vi "Configuration Window.vi"(8 "error in (no error)":errorcluster, 11 "Inst.RP100 in":refnum<class "Inst.RP100.lvclass">) -> (0 "error out":errorcluster, 3 "Inst.RP100 out":refnum<class "Inst.RP100.lvclass">)   [LabVIEW 2019, in "Inst.RP100.lvlib" / "Inst.RP100.lvclass"]
uses:
  Inst.RP100.lvclass
  C:/Program Files (x86)/National Instruments/LabVIEW 2019/user.lib/LevyLab/Instrument Framework/Instrument/Instrument.lvclass
  <userlib>/LevyLab/Instrument Framework/Instrument/Instrument.lvclass/Instrument.ctl
  <userlib>/LevyLab/Instrument Framework/Instrument/Instrument.lvclass
  C:/Program Files (x86)/National Instruments/LabVIEW 2019/user.lib/LevyLab/Instrument Framework/Instrument Types/Strain/Instrument.Strain.lvclass
  C:/Program Files (x86)/National Instruments/LabVIEW 2019/vi.lib/JKI/JKI SMO/SMO/SMO.lvclass
panel:
  in  "Cancel":bool
  in  "RP100 Address":refnum<visa-resource-name>
  in  "OK":bool
  # "Confirm or Make Changes:"
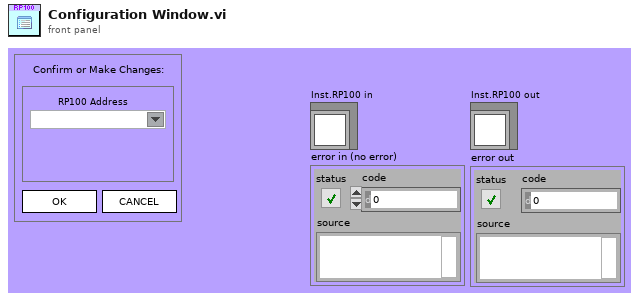
[diagram p1: front panel]
types:
  T1 = enum32{"Invalid", "Standard", "Closed", "Hidden", "Minimized", "Maximized"}
  T2 = enum32{"invalid app kind", "Development System", "Run Time System", "Student Edition", "Embedded LabVIEW", "Evaluation", "Custom"}
  T3 = cluster{"Core":cluster{"Current VI Reference":refnum<vi>, "Close Panel on Exit?":bool}, "Address":string}
  T4 = cluster{"Current VI Reference":refnum<vi>, "Close Panel on Exit?":bool}
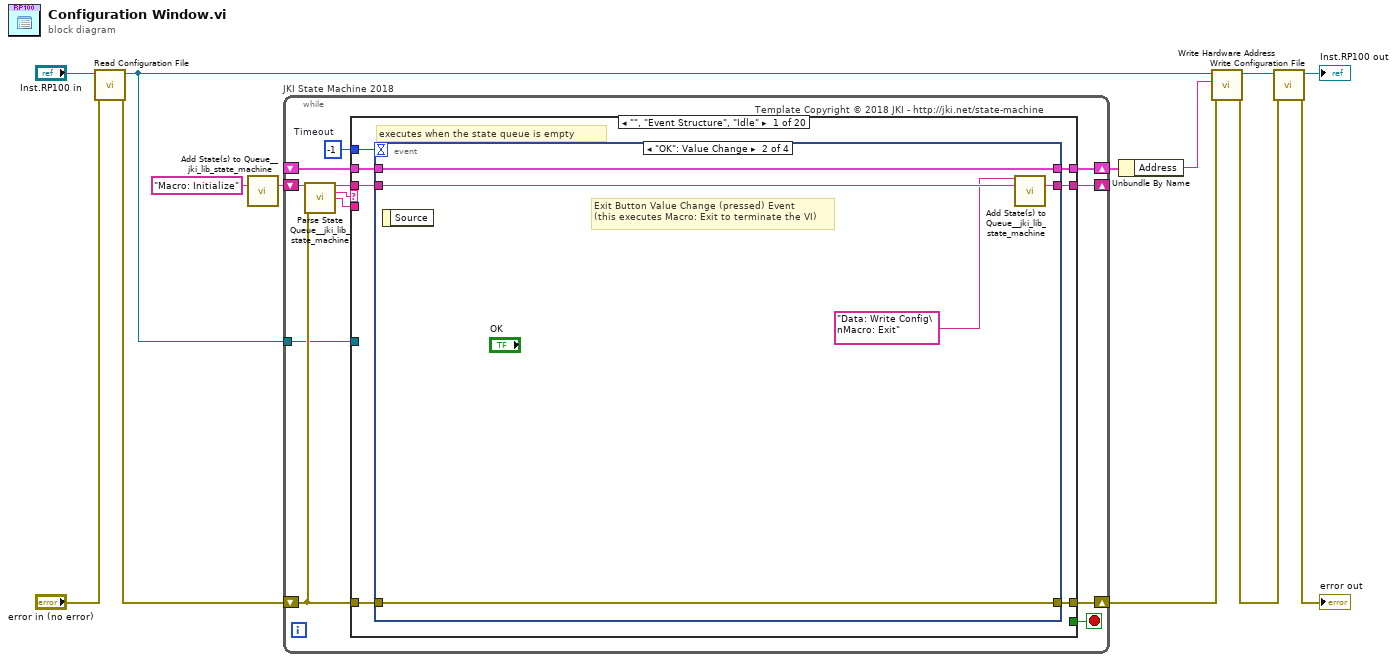
[diagram p0: block diagram]
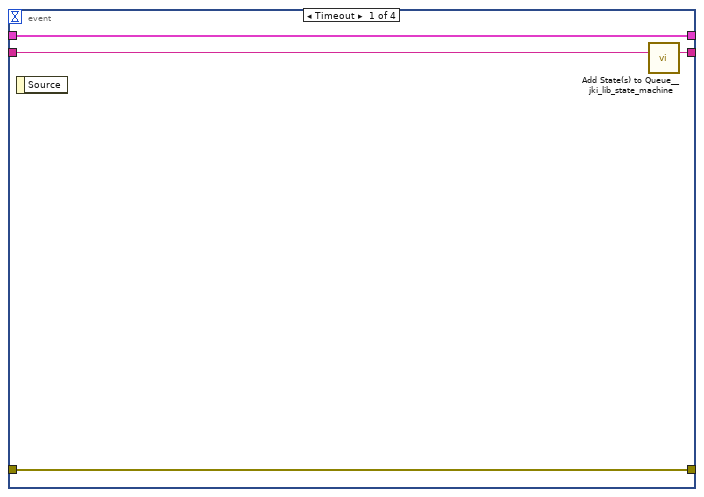
[diagram p2: hidden frame]
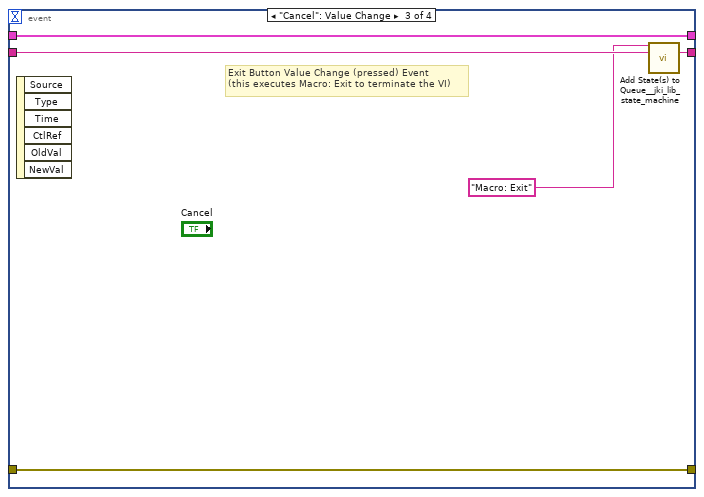
[diagram p3: hidden frame]
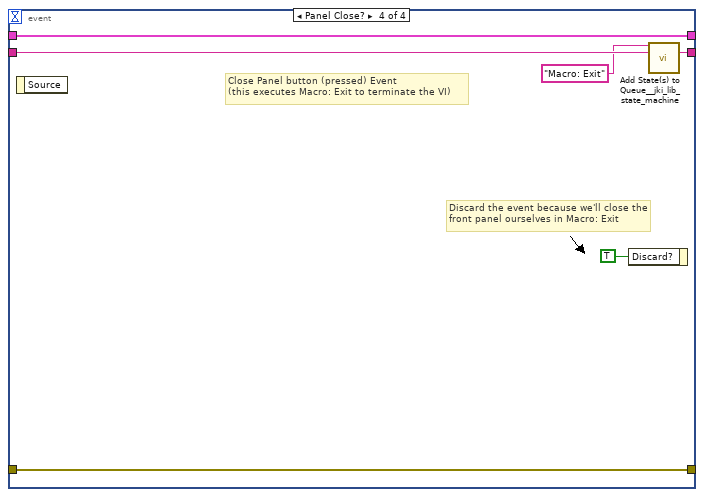
[diagram p4: hidden frame]
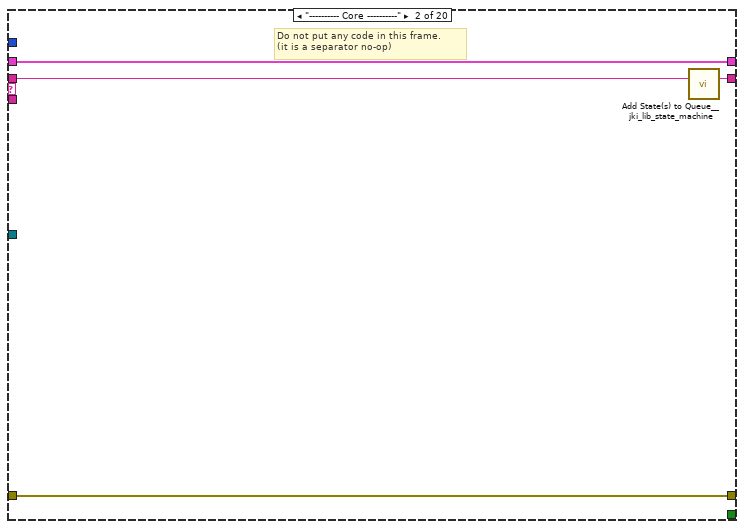
[diagram p5: hidden frame]
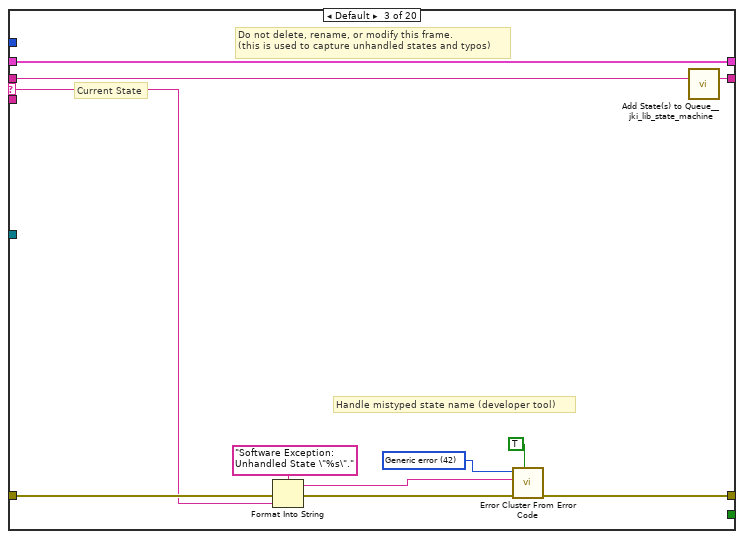
[diagram p6: hidden frame]
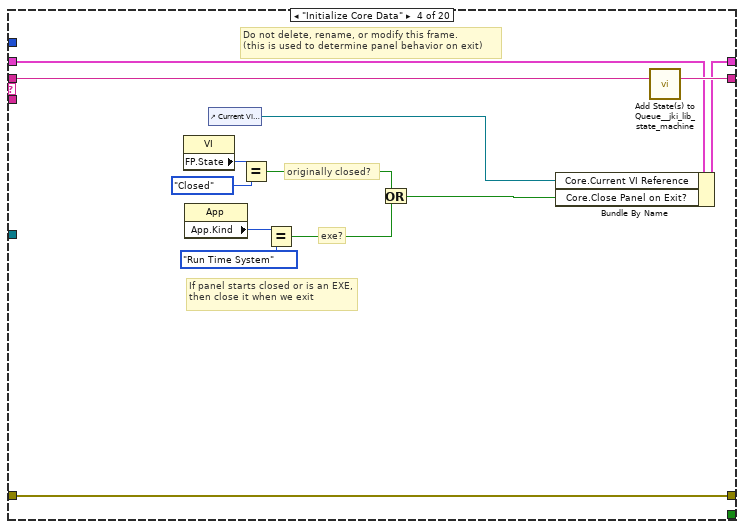
[diagram p7: hidden frame]
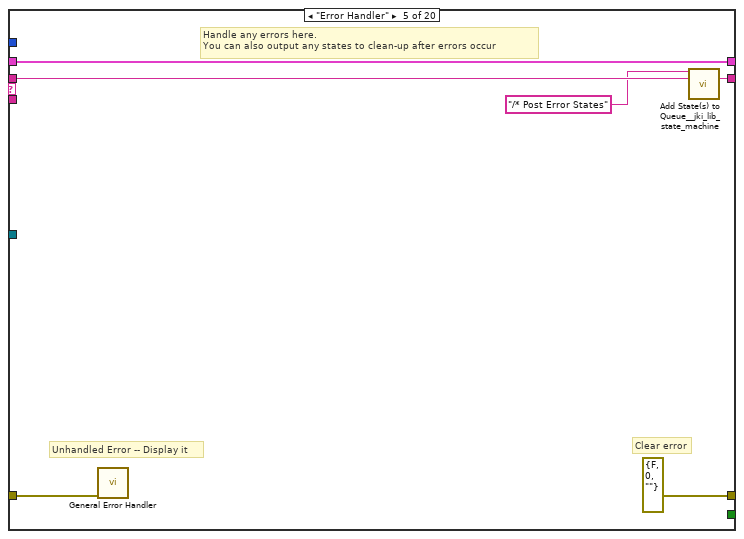
[diagram p8: hidden frame]
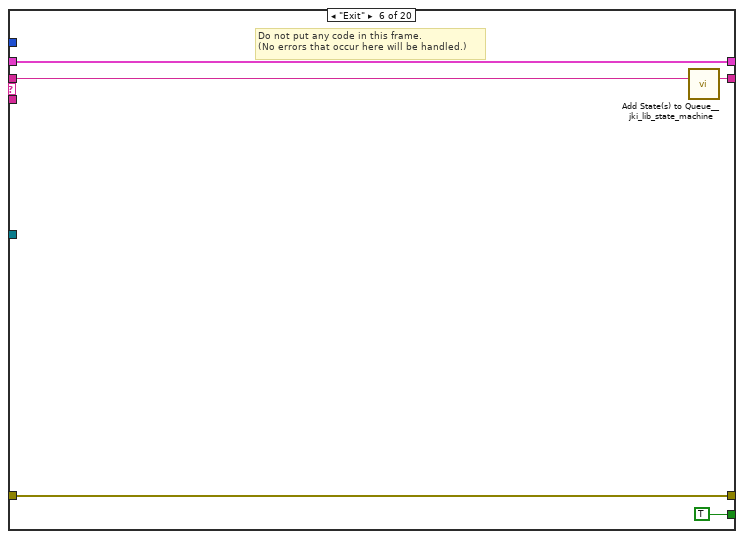
[diagram p9: hidden frame]
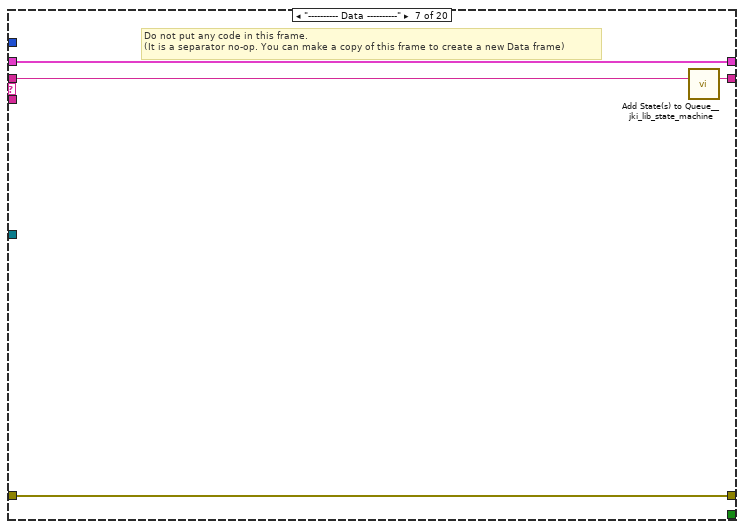
[diagram p10: hidden frame]
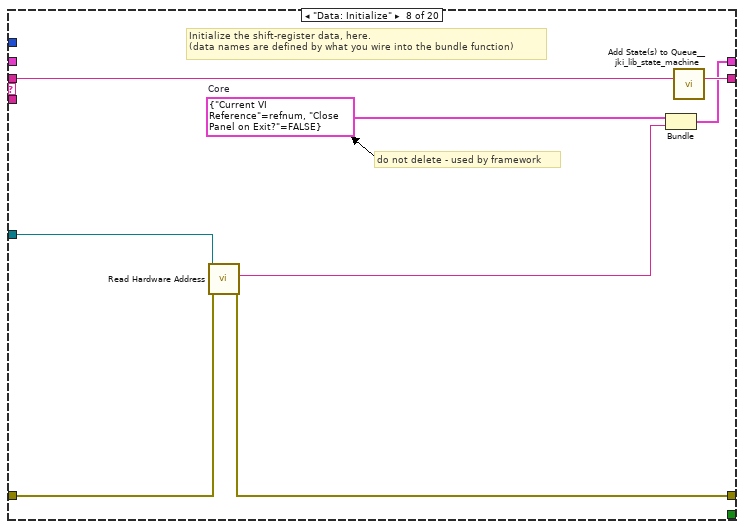
[diagram p11: hidden frame]
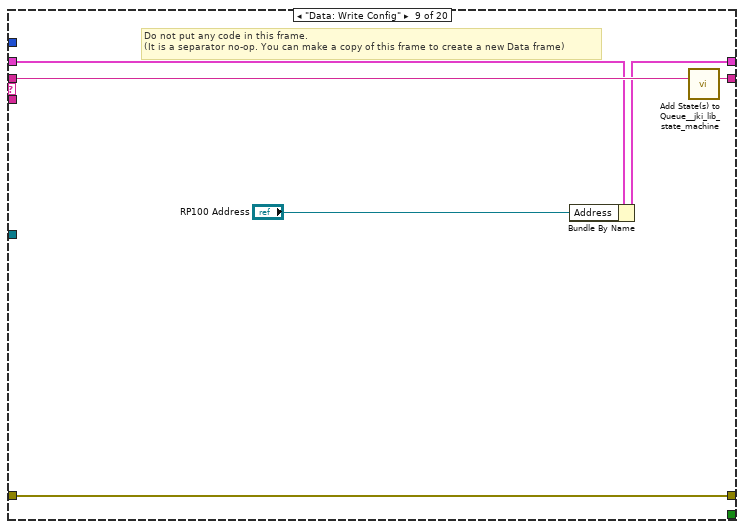
[diagram p12: hidden frame]
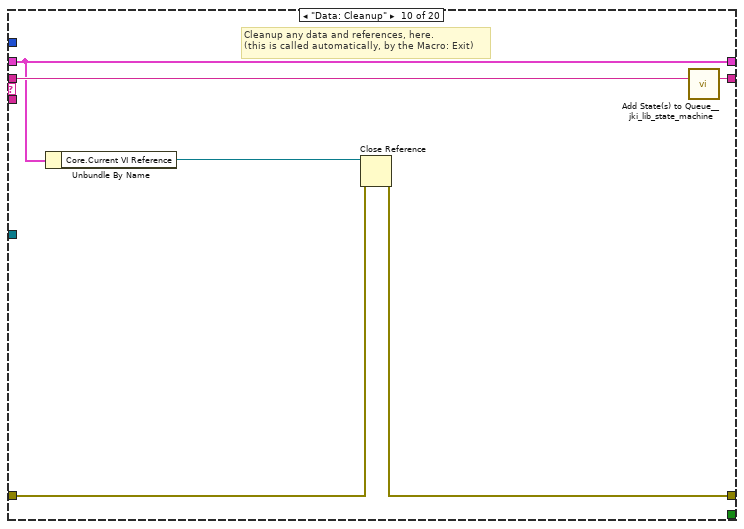
[diagram p13: hidden frame]
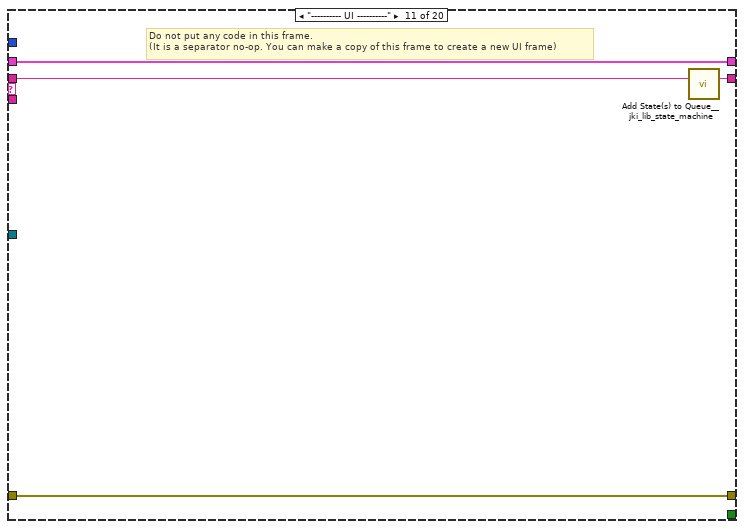
[diagram p14: hidden frame]
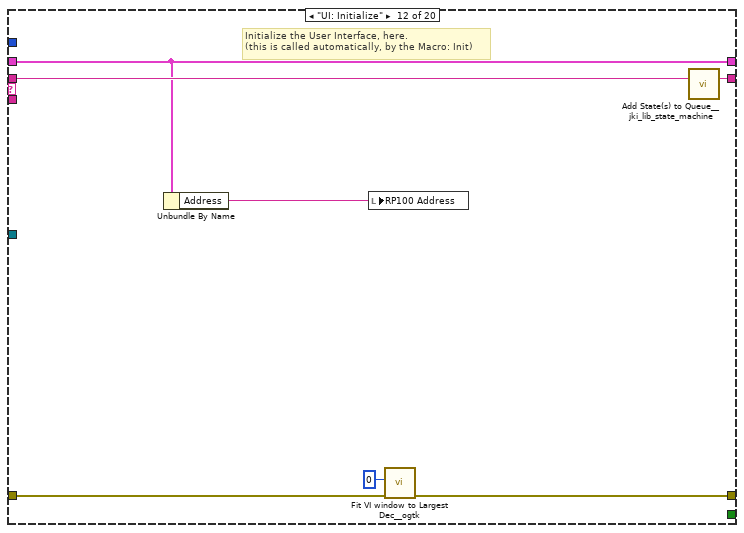
[diagram p15: hidden frame]
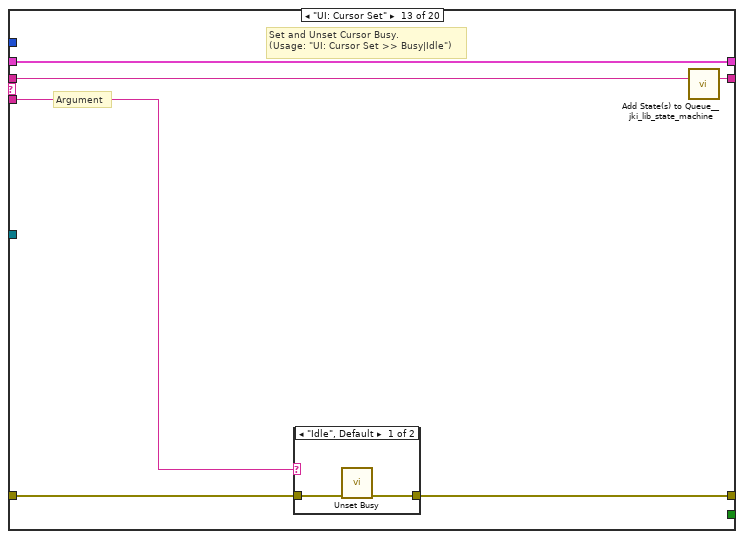
[diagram p16: hidden frame]
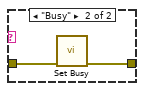
[diagram p17: hidden frame]
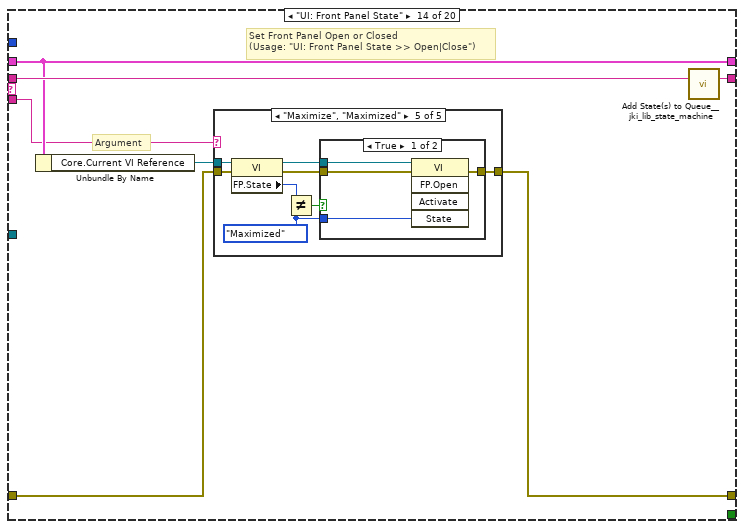
[diagram p18: hidden frame]
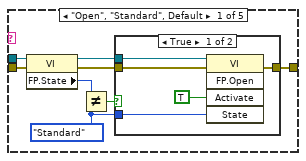
[diagram p19: hidden frame]
diagram:
  n1 = call-dynamic "Read Configuration File.vi"("error in (no error)"="error in (no error)", "Inst.RP100 in"="Inst.RP100 in") -> ("error out"=w8:errorcluster, "Inst.RP100 out"=w6:refnum<class "Inst.RP100.lvclass">)  [unwired: 8 in]
  n2 = call <vilib>:"Add State(s) to Queue__jki_lib_state_machine.vi"("State(s) in (\"\")"="Macro: Initialize") -> ("States Out"=w13:string)  [unwired: 14 in]
  n3 = while "JKI State Machine 2018" {
    shift-right: [w18] -> w2
    shift-left: _ -> [w17]
    shift-right: [w21] -> w4
    shift-left: w8 -> [w15]
    shift-right: [w20] -> _
    shift-left: w13 -> [w22]
    tunnel: w6 -> [w14]
    stop <- w19 stop-if-true
    w16 = -1  # Timeout
    # "Template Copyright © 2018 JKI - http://jki.net/state-machine"
    n4 = call <vilib>:"Parse State Queue__jki_lib_state_machine.vi"("State Queue"=w22, "Error In (no error)"=w15) -> ("Remaining States"=w24:string, "Current State"=w25:string, "Arguments"=w23:string)  [unwired: 11 in]
    n5 = case shown="\"\", \"Event Structure\", \"Idle\"" w25 {
      selector: w25 -> [_ _ w57 _ _ _ _ _ _ _ _ _ _ _ _ _ _ _ _ _]
      tunnel: w24 -> [w32 w56 w61 w80 w86 w91 w95 w103 w109 w115 w119 w126 w132 w143 w212 w217 w227 w231 w235 w239]
      tunnel: w23 -> [_ _ _ _ _ _ _ _ _ _ _ _ w127 w137 _ _ _ _ _ _]
      tunnel: w17 -> [w30 w53 w59 w73 w83 w89 w92 _ w106 w110 w116 w121 w130 w139 w209 w214 w224 w228 w232 w236]
      tunnel: [w29 w54 w63 w77 errorcluster {"status"=FALSE, "code"=0, "source"=""} ("error out") w88 w93 w97 w104 w111 w117 w124 w128 w140 w210 w215 w225 w229 w233 w237] -> w21
      tunnel: w15 -> [w28 w54 w62 w77 w82 w88 w93 w96 w104 w112 w117 w123 w129 w141 w210 w215 w225 w229 w233 w237]
      tunnel: [w31 w55 w60 w79 w85 w90 w94 w102 w108 w114 w118 w125 w131 w142 w211 w216 w226 w230 w234 w238] -> w20
      tunnel: [_ _ _ _ _ TRUE _ _ _ _ _ _ _ _ _ _ _ _ _ _] -> w19
      tunnel: [w27 w53 w59 w78 w83 w89 w92 w101 w107 w110 w116 w121 w130 w139 w209 w214 w224 w228 w232 w236] -> w18
      tunnel: w16 -> [w26 _ _ _ _ _ _ _ _ _ _ _ _ _ _ _ _ _ _ _]
      tunnel: w14 -> [_ _ _ _ _ _ _ w99 _ _ _ _ _ _ _ _ _ _ _ _]
      frame "", "Event Structure", "Idle" {
        # "executes when the state queue is empty"
        n6 = event shown="[1] \"OK\": Value Change" {
          selector: _ -> [_ _ _ _]
          dyn-events: _ -> [_ _ _ _]
          timeout: w26 -> [_ _ _ _]
          tunnel: w32 -> [w36 w41 w46 w52]
          tunnel: [w35 w40 w45 w51] -> w31
          tunnel: w30 -> [w33 w38 w43 w49]
          tunnel: [w34 w39 w44 w50] -> w29
          tunnel: w28 -> [w34 w39 w44 w50]
          tunnel: [w33 w38 w43 w49] -> w27
          event Timeout {
            n7 = event-data() -> ()  [unwired: 1 in, 1 out]
            n8 = call <vilib>:"Add State(s) to Queue__jki_lib_state_machine.vi"("State(s) in (\"\")"=w36) -> ("States Out"=w35:string)  [unwired: 14 in]
          }
          event "OK": Value Change {
            # "Exit Button Value Change (pressed) Event\n(this executes Macro: Exit to terminate the VI)"
            n9 = event-data() -> ()  [unwired: 1 in, 1 out]
            n10 = call <vilib>:"Add State(s) to Queue__jki_lib_state_machine.vi"("State(s) in Front (\"\")"="Data: Write Config\nMacro: Exit", "State(s) in (\"\")"=w41) -> ("States Out"=w40:string)  [unwired: 13 in]
          }
          event "Cancel": Value Change {
            # "Exit Button Value Change (pressed) Event\n(this executes Macro: Exit to terminate the VI)"
            n11 = event-data() -> ()  [unwired: 1 in, 6 out]
            n12 = call <vilib>:"Add State(s) to Queue__jki_lib_state_machine.vi"("State(s) in Front (\"\")"="Macro: Exit", "State(s) in (\"\")"=w46) -> ("States Out"=w45:string)  [unwired: 13 in]
          }
          event Panel Close? {
            # "Discard the event because we'll close the front panel ourselves in Macro: Exit"
            # "Close Panel button (pressed) Event\n(this executes Macro: Exit to terminate the VI)"
            n13 = event-data() -> ()  [unwired: 1 in, 1 out]
            n14 = event-data("Discard?"=TRUE) -> ()  [unwired: 1 in, 1 out]
            n15 = call <vilib>:"Add State(s) to Queue__jki_lib_state_machine.vi"("State(s) in Front (\"\")"="Macro: Exit", "State(s) in (\"\")"=w52) -> ("States Out"=w51:string)  [unwired: 13 in]
          }
        }
      }
      frame "---------- Core ----------" {
        # "Do not put any code in this frame.\n(it is a separator no-op)"
        n16 = call <vilib>:"Add State(s) to Queue__jki_lib_state_machine.vi"("State(s) in (\"\")"=w56) -> ("States Out"=w55:string)  [unwired: 14 in]
      }
      frame Default {
        w66 = 42 items=["No error", "Argument error", "Memory is full", "Out of zone", "End of file", "File already open", "Generic file I/O error", "File not found", "File permission error", "Disk is full", "Duplicate path", "Too many files open", "System feature not enabled", "Resource file not found", "Cannot add resource", "Resource not found", "Image not found", "Image memory error", "Pen does not exist", "Config type invalid", "Config token not found", "Config parse error", "Config memory error", "Bad external code format", "Bad external code offset", "External code not present", "Null window", "Destroy window error", "Null menu", "Print aborted", "Bad print record", "Print driver error", "Windows error during printing", "Memory error during printing", "Print dialog error", "Generic print error", "Invalid device refnum", "Device not found", "Device parameter error", "Device unit error", "Cannot open device", "Device call aborted", "Generic error", "Cancelled by user", "Object ID too low", "Object ID too high", "Object not in heap", "Unknown heap", "Unknown object (invalid DefProc)", "Unknown object (DefProc not in table)", "Message out of range", "Invalid (null) method", "Unknown message", "Manager call not supported", "Bad address", "Network operation in progress", "Network operation timed out", "Connection is busy", "Network attribute not supported", "Network error", "Address in use", "System out of memory", "Connection aborted", "Connection refused", "Not connected", "Already connected", "Connection closed", "Initialization error (interapplication manager)", "Bad occurrence", "Wait on unbound occurrence handler", "Occurrence queue overflow", "Datalog type conflict", "Unused", "Unrecognized type (interapplication manager)", "Memory corrupt", "Failed to make temporary DLL", "Old CIN version", "Drag socket not found", "Failed to load drop-object", "Failed to register OLE object", "Failed to release OLE object", "Format specifier type mismatch", "Unknown format specifier", "Too few format specifiers", "Too many format specifiers", "Scan failed", "Newer CIN version", "Error converting to variant", "Runtime menu error", "Password tampered", "Variant attribute not found", "Incompatible variant data type", "Event data is not available", "Event Store is not present", "Occurrence is not found", "Event Queue is not created", "Event info is not available", "Refnum passed is NULL", "Error retrieving Class GUID", "Error retrieving CoClass GUID", "Error retrieving TypeLib GUID.", "Bad built application magic bytes.", "Specific driver is different from the specific driver associated with the Logical Name.", "There is no session opened to the class driver.", "Max Error", "MAX - Error with config objects", "MAX - Error loading configuration", "MAX - Group not supported"]
        # "Current State"
        # "Do not delete, rename, or modify this frame.\n(this is used to capture unhandled states and typos)"
        # "Handle mistyped state name (developer tool)"
        n17 = Format Into String(format string="Software Exception: Unhandled State \"%s\"." ("message"), error in=w62, w57) -> (resulting string=w65:string, error out=w64:errorcluster)  [unwired: 1 in]
        n18 = call <vilib>:"Error Cluster From Error Code.vi"("show call chain? (False)"=TRUE, "error in (no error)"=w64, "error message (\"\")"=w65, "error code (0)"=w66) -> ("error out"=w63:errorcluster)  [unwired: 5 in]
        n19 = call <vilib>:"Add State(s) to Queue__jki_lib_state_machine.vi"("State(s) in (\"\")"=w61) -> ("States Out"=w60:string)  [unwired: 14 in]
      }
      frame "Initialize Core Data" {
        # "Do not delete, rename, or modify this frame.\n(this is used to determine panel behavior on exit)"
        # "originally closed?"
        # "exe?"
        # "If panel starts closed or is an EXE, then close it when we exit"
        n20 = property class="VI"() -> ("FP.State"=w70:T1)  [unwired: 2 in, 2 out]
        n21 = property class="App"() -> ("App.Kind"=w76:T2)  [unwired: 2 in, 2 out]
        n22 = control-ref of="Current VI Reference"() -> (w71:refnum<vi>)
        n23 = Equal?(x=w70, y=T1."Closed" ("Front Panel Window:State")) -> (x = y?=w68:bool)
        n24 = Equal?(x=w76, y=T2."Run Time System" ("Application:Kind")) -> (x = y?=w74:bool)
        n25 = Or(x=w68, y=w74) -> (x .or. y?=w72:bool)
        n26 = Bundle By Name(cluster=w73, "Core.Current VI Reference"=w71, "Core.Close Panel on Exit?"=w72) -> (w78:T3)
        n27 = call <vilib>:"Add State(s) to Queue__jki_lib_state_machine.vi"("State(s) in (\"\")"=w80) -> ("States Out"=w79:string)  [unwired: 14 in]
      }
      frame "Error Handler" {
        # "Unhandled Error -- Display it"
        # "Handle any errors here.\nYou can also output any states to clean-up after errors occur"
        # "Clear error"
        n28 = call <vilib>:"General Error Handler.vi"("error in (no error)"=w82) -> ()  [unwired: 10 in, 5 out]
        n29 = call <vilib>:"Add State(s) to Queue__jki_lib_state_machine.vi"("State(s) in Front (\"\")"="/* Post Error States", "State(s) in (\"\")"=w86) -> ("States Out"=w85:string)  [unwired: 13 in]
      }
      frame "Exit" {
        # "Do not put any code in this frame.\n(No errors that occur here will be handled.)"
        n30 = call <vilib>:"Add State(s) to Queue__jki_lib_state_machine.vi"("State(s) in (\"\")"=w91) -> ("States Out"=w90:string)  [unwired: 14 in]
      }
      frame "---------- Data ----------" {
        # "Do not put any code in this frame.\n(It is a separator no-op. You can make a copy of this frame to create a new Data frame)"
        n31 = call <vilib>:"Add State(s) to Queue__jki_lib_state_machine.vi"("State(s) in (\"\")"=w95) -> ("States Out"=w94:string)  [unwired: 14 in]
      }
      frame "Data: Initialize" {
        w100 = T4 {"Current VI Reference"=refnum, "Close Panel on Exit?"=FALSE}  # Core
        # "do not delete - used by framework"
        # "Initialize the shift-register data, here.\n(data names are defined by what you wire into the bundle function)"
        n32 = call <userlib>:"Read Hardware Address.vi"("error in (no error)"=w96, "Instrument in"=w99) -> ("error out"=w97:errorcluster, "Address"=w98:string)  [unwired: 7 in, 1 out]
        n33 = Bundle("Core"=w100, "Address"=w98) -> (w101:T3)  [unwired: 1 in]
        n34 = call <vilib>:"Add State(s) to Queue__jki_lib_state_machine.vi"("State(s) in (\"\")"=w103) -> ("States Out"=w102:string)  [unwired: 14 in]
      }
      frame "Data: Write Config" {
        # "Do not put any code in this frame.\n(It is a separator no-op. You can make a copy of this frame to create a new Data frame)"
        n35 = Bundle By Name(cluster=w106, "Address"="RP100 Address") -> (w107:T3)
        n36 = call <vilib>:"Add State(s) to Queue__jki_lib_state_machine.vi"("State(s) in (\"\")"=w109) -> ("States Out"=w108:string)  [unwired: 14 in]
      }
      frame "Data: Cleanup" {
        # "Cleanup any data and references, here.\n(this is called automatically, by the Macro: Exit)"
        n37 = Unbundle By Name(w110) -> ("Core.Current VI Reference"=w113:refnum<vi>)
        n38 = Close Reference(reference=w113, error in (no error)=w112) -> (error out=w111:errorcluster)
        n39 = call <vilib>:"Add State(s) to Queue__jki_lib_state_machine.vi"("State(s) in (\"\")"=w115) -> ("States Out"=w114:string)  [unwired: 14 in]
      }
      frame "---------- UI ----------" {
        # "Do not put any code in this frame.\n(It is a separator no-op. You can make a copy of this frame to create a new UI frame)"
        n40 = call <vilib>:"Add State(s) to Queue__jki_lib_state_machine.vi"("State(s) in (\"\")"=w119) -> ("States Out"=w118:string)  [unwired: 14 in]
      }
      frame "UI: Initialize" {
        # "Initialize the User Interface, here.\n(this is called automatically, by the Macro: Init)"
        n41 = Unbundle By Name(w121) -> ("Address"=w120:string)
        n42 = local write "RP100 Address"(w120) -> ()
        n43 = call <userlib>:"Fit VI window to Largest Dec__ogtk.vi"("error in (no error)"=w123, "border spacing (2 px)"=0) -> ("error out"=w124:errorcluster)  [unwired: 4 in, 1 out]
        n44 = call <vilib>:"Add State(s) to Queue__jki_lib_state_machine.vi"("State(s) in (\"\")"=w126) -> ("States Out"=w125:string)  [unwired: 14 in]
      }
      frame "UI: Cursor Set" {
        # "Argument"
        # "Set and Unset Cursor Busy.\n(Usage: \"UI: Cursor Set >> Busy|Idle\")"
        n45 = case shown="\"Idle\", Default" w127 {
          tunnel: w129 -> [w134 w136]
          tunnel: [w133 w135] -> w128
          frame "Idle", Default {
            n46 = call <vilib>:"Unset Busy.vi"("error in (no error)"=w134) -> ("error out"=w133:errorcluster)  [unwired: 10 in]
          }
          frame "Busy" {
            n47 = call <vilib>:"Set Busy.vi"("error in (no error)"=w136) -> ("error out"=w135:errorcluster)  [unwired: 9 in, 1 out]
          }
        }
        n48 = call <vilib>:"Add State(s) to Queue__jki_lib_state_machine.vi"("State(s) in (\"\")"=w132) -> ("States Out"=w131:string)  [unwired: 14 in]
      }
      frame "UI: Front Panel State" {
        # "Argument"
        # "Set Front Panel Open or Closed\n(Usage: \"UI: Front Panel State >> Open|Close\")"
        n49 = Unbundle By Name(w139) -> ("Core.Current VI Reference"=w138:refnum<vi>)
        n50 = case shown="\"Maximize\", \"Maximized\"" w137 {
          tunnel: w141 -> [w149 w164 w175 w188 w201]
          tunnel: [w151 w165 w177 w190 w203] -> w140
          tunnel: w138 -> [w150 w162 w176 w189 w202]
          frame "Open", "Standard", Default {
            w144 = T1."Standard" ("State")
            n51 = property class="VI"(reference=w150, error in=w149) -> (reference out=w147:refnum<vi>, error out=w148:errorcluster, "FP.State"=w146:T1)
            n52 = Not Equal?(x=w146, y=w144) -> (x != y?=w145:bool)
            n53 = case shown="True" w145 {
              tunnel: [w155 w157] -> w151
              tunnel: w148 -> [w154 w157]
              tunnel: w147 -> [w153 _]
              tunnel: w144 -> [w152 _]
              frame True {
                n54 = invoke class="VI" method="FP.Open"(reference=w153, error in=w154, "Activate"=TRUE, "State"=w152) -> (error out=w155:errorcluster)  [unwired: 1 in, 4 out]
              }
              frame False {
              }
            }
          }
          frame "Close", "Closed" {
            n55 = property class="VI"(reference=w162, error in=w164) -> (reference out=w161:refnum<vi>, error out=w163:errorcluster, "FP.State"=w159:T1)
            n56 = Not Equal?(x=w159, y=T1."Closed" ("Front Panel Window:State")) -> (x != y?=w158:bool)
            n57 = case shown="True" w158 {
              tunnel: [w166 w169] -> w165
              tunnel: w163 -> [w166 w168]
              tunnel: w161 -> [_ w167]
              frame False {
              }
              frame True {
                n58 = invoke class="VI" method="FP.Close"(reference=w167, error in=w168) -> (error out=w169:errorcluster)  [unwired: 1 in, 2 out]
              }
            }
          }
          frame "Hidden", "Hide" {
            w170 = T1."Hidden" ("State")
            n59 = property class="VI"(reference=w176, error in=w175) -> (reference out=w173:refnum<vi>, error out=w174:errorcluster, "FP.State"=w172:T1)
            n60 = Not Equal?(x=w172, y=w170) -> (x != y?=w171:bool)
            n61 = case shown="True" w171 {
              tunnel: [w181 w182] -> w177
              tunnel: w174 -> [w180 w182]
              tunnel: w173 -> [w179 _]
              tunnel: w170 -> [w178 _]
              frame True {
                n62 = invoke class="VI" method="FP.Open"(reference=w179, error in=w180, "State"=w178) -> (error out=w181:errorcluster)  [unwired: 2 in, 4 out]
              }
              frame False {
              }
            }
          }
          frame "Minimize", "Minimized" {
            w183 = T1."Minimized" ("State")
            n63 = property class="VI"(reference=w189, error in=w188) -> (reference out=w186:refnum<vi>, error out=w187:errorcluster, "FP.State"=w185:T1)
            n64 = Not Equal?(x=w185, y=w183) -> (x != y?=w184:bool)
            n65 = case shown="True" w184 {
              tunnel: [w194 w195] -> w190
              tunnel: w187 -> [w193 w195]
              tunnel: w186 -> [w192 _]
              tunnel: w183 -> [w191 _]
              frame True {
                n66 = invoke class="VI" method="FP.Open"(reference=w192, error in=w193, "State"=w191) -> (error out=w194:errorcluster)  [unwired: 2 in, 4 out]
              }
              frame False {
              }
            }
          }
          frame "Maximize", "Maximized" {
            w196 = T1."Maximized" ("State")
            n67 = property class="VI"(reference=w202, error in=w201) -> (reference out=w199:refnum<vi>, error out=w200:errorcluster, "FP.State"=w198:T1)
            n68 = Not Equal?(x=w198, y=w196) -> (x != y?=w197:bool)
            n69 = case shown="True" w197 {
              tunnel: [w207 w208] -> w203
              tunnel: w200 -> [w206 w208]
              tunnel: w199 -> [w205 _]
              tunnel: w196 -> [w204 _]
              frame True {
                n70 = invoke class="VI" method="FP.Open"(reference=w205, error in=w206, "State"=w204) -> (error out=w207:errorcluster)  [unwired: 2 in, 4 out]
              }
              frame False {
              }
            }
          }
        }
        n71 = call <vilib>:"Add State(s) to Queue__jki_lib_state_machine.vi"("State(s) in (\"\")"=w143) -> ("States Out"=w142:string)  [unwired: 14 in]
      }
      frame "---------- Macro ----------" {
        # "Do not put any code in this frame.\n(It is a separator no-op. You can make a copy of this frame to create a new Macro frame)"
        n72 = call <vilib>:"Add State(s) to Queue__jki_lib_state_machine.vi"("State(s) in (\"\")"=w212) -> ("States Out"=w211:string)  [unwired: 14 in]
      }
      frame "Macro: Initialize" {
        w213 = "Data: Initialize\nInitialize Core Data\nUI: Initialize\nUI: Front Panel State >> Open"  # Data: Initialize Initialize Core Data UI: Initialize UI: Front Panel State >> Open
        # "Initialization Macro\n(This is called once, when the VI starts)"
        n73 = call <vilib>:"Add State(s) to Queue__jki_lib_state_machine.vi"("State(s) in Front (\"\")"=w213, "State(s) in (\"\")"=w217) -> ("States Out"=w216:string)  [unwired: 13 in]
      }
      frame "Macro: Exit" {
        # "Exit Macro\n(This is called once, when the VI exits)"
        n74 = Unbundle By Name(w224) -> ("Core.Close Panel on Exit?"=w223:bool)
        n75 = Select(t="UI: Front Panel State >> Close", s=w223, f="" ("Empty String Constant")) -> (s? t:f=w220:string)
        n76 = call <vilib>:"Add State(s) to Queue__jki_lib_state_machine.vi"("State(s) in (\"\")"=w220, "State(s) at Back (\"\")"="Data: Cleanup\nExit") -> ("States Out"=w218:string)  [unwired: 13 in]
        n77 = call <vilib>:"Add State(s) to Queue__jki_lib_state_machine.vi"("State(s) in Front (\"\")"=w218, "State(s) in (\"\")"=w227) -> ("States Out"=w226:string)  [unwired: 13 in]
      }
      frame "---------- New Category ----------" {
        # "Template Separator\n(You can make a copy of, or modify, this frame)"
        n78 = call <vilib>:"Add State(s) to Queue__jki_lib_state_machine.vi"("State(s) in (\"\")"=w231) -> ("States Out"=w230:string)  [unwired: 14 in]
      }
      frame "New Category: 1" {
        # "Your code here.\n(You can make a copy of, or modify, this frame)"
        n79 = call <vilib>:"Add State(s) to Queue__jki_lib_state_machine.vi"("State(s) in (\"\")"=w235) -> ("States Out"=w234:string)  [unwired: 14 in]
      }
      frame "New Category: 2" {
        # "Your code here.\n(You can make a copy of, or modify, this frame)"
        n80 = call <vilib>:"Add State(s) to Queue__jki_lib_state_machine.vi"("State(s) in (\"\")"=w239) -> ("States Out"=w238:string)  [unwired: 14 in]
      }
    }
  }
  n81 = Unbundle By Name(w2) -> ("Address"=w1:string)
  n82 = call <userlib>:"Write Hardware Address.vi"("error in (no error)"=w4, "Address"=w1, "Instrument in"=w6) -> ("error out"=w3:errorcluster, "Instrument out"=w5:refnum<class "Inst.RP100.lvclass">)  [unwired: 7 in]
  n83 = call-dynamic "Write Configuration File.vi"("error in (no error)"=w3, "Inst.RP100 in"=w5) -> ("error out"=→"error out":errorcluster, "Inst.RP100 out"=→"Inst.RP100 out":refnum<class "Inst.RP100.lvclass">)  [unwired: 8 in]
